vi "Import File - Tx Packet XML.vi"(6 "Root Node":refnum<k24>, 8 "error in (no error)":errorcluster) -> (0 "error out":errorcluster, 1 "Packet Header Data":T6, 4 "Tx Packet":T1 {"Endianness" items=["big-endian"=0, "little-endian"=2]})   [LabVIEW 2016, in "UDP-Custom-Device System Explorer.lvlib"]
uses:
  UDP-Custom-Device System Explorer.lvlib
  System.Xml
  Types/XML - New/ImpExp - Packet Headers.ctl
  Types/XML - New/ImpExp - Tx Packet Data.ctl
  <vilib>/NI Veristand/Custom Device API/Custom Device Item Info.ctl
  Shared/Types/Shared - Channel Data Type.ctl
  Shared/Types/Shared - Buffered.PacketInfo.ctl
  Shared/Types/Shared - Pointer Encoding.ctl
  <vilib>/NI VeriStand/Custom Device API/Custom Device API.lvlib
  Shared/UDP-Custom-Device Shared.lvlib
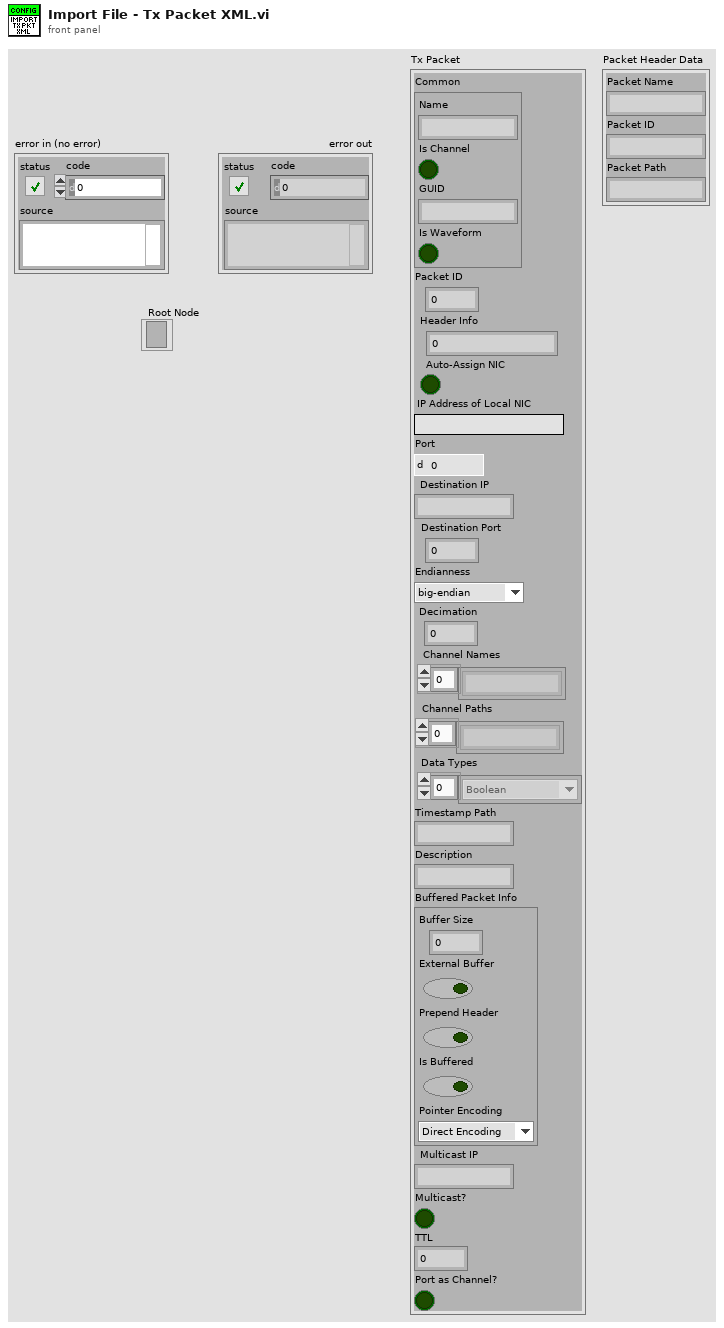
[diagram p1: front panel]
types:
  T1 = typedef "UDP-Custom-Device System Explorer.lvlib/ImpExp - Tx Packet Data.ctl" = cluster{"Common":T2, "Packet ID":i32, "Header Info":u32, "Auto-Assign NIC":bool, "IP Address of Local NIC":string, "Port":u16, "Destination IP":string, "Destination Port":u16, "Endianness":u16, "Decimation":u16, "Channel Names":string[], "Channel Paths":string[], "Data Types":T3[], "Timestamp Path":string, "Description":string, "Buffered Packet Info":T4, "Multicast IP":string, "Multicast?":bool, "TTL":u16, "Port as Channel?":bool}
  T2 = typedef "Custom Device API.lvlib/Custom Device Item Info.ctl" = cluster{"Name":string, "Is Channel":bool, "GUID":string, "Is Waveform":bool}
  T3 = typedef "UDP-Custom-Device Shared.lvlib/Shared - Channel Data Type.ctl" = enum16{"Boolean", "Single", "Double", "I8", "I16", "I32", "I64", "U8", "U16", "U32", "U64"}
  T4 = typedef "UDP-Custom-Device Shared.lvlib/Shared - Buffered.PacketInfo.ctl" = cluster{"Buffer Size":i32, "External Buffer":bool, "Prepend Header":bool, "Is Buffered":bool, "Pointer Encoding":T5}
  T5 = typedef "UDP-Custom-Device Shared.lvlib/Shared - Pointer Encoding.ctl" = enum16{"Direct Encoding", "Conversion Encoding"}
  T6 = typedef "UDP-Custom-Device System Explorer.lvlib/ImpExp - Packet Headers.ctl" = cluster{"Packet Name":string, "Packet ID":string, "Packet Path":string}
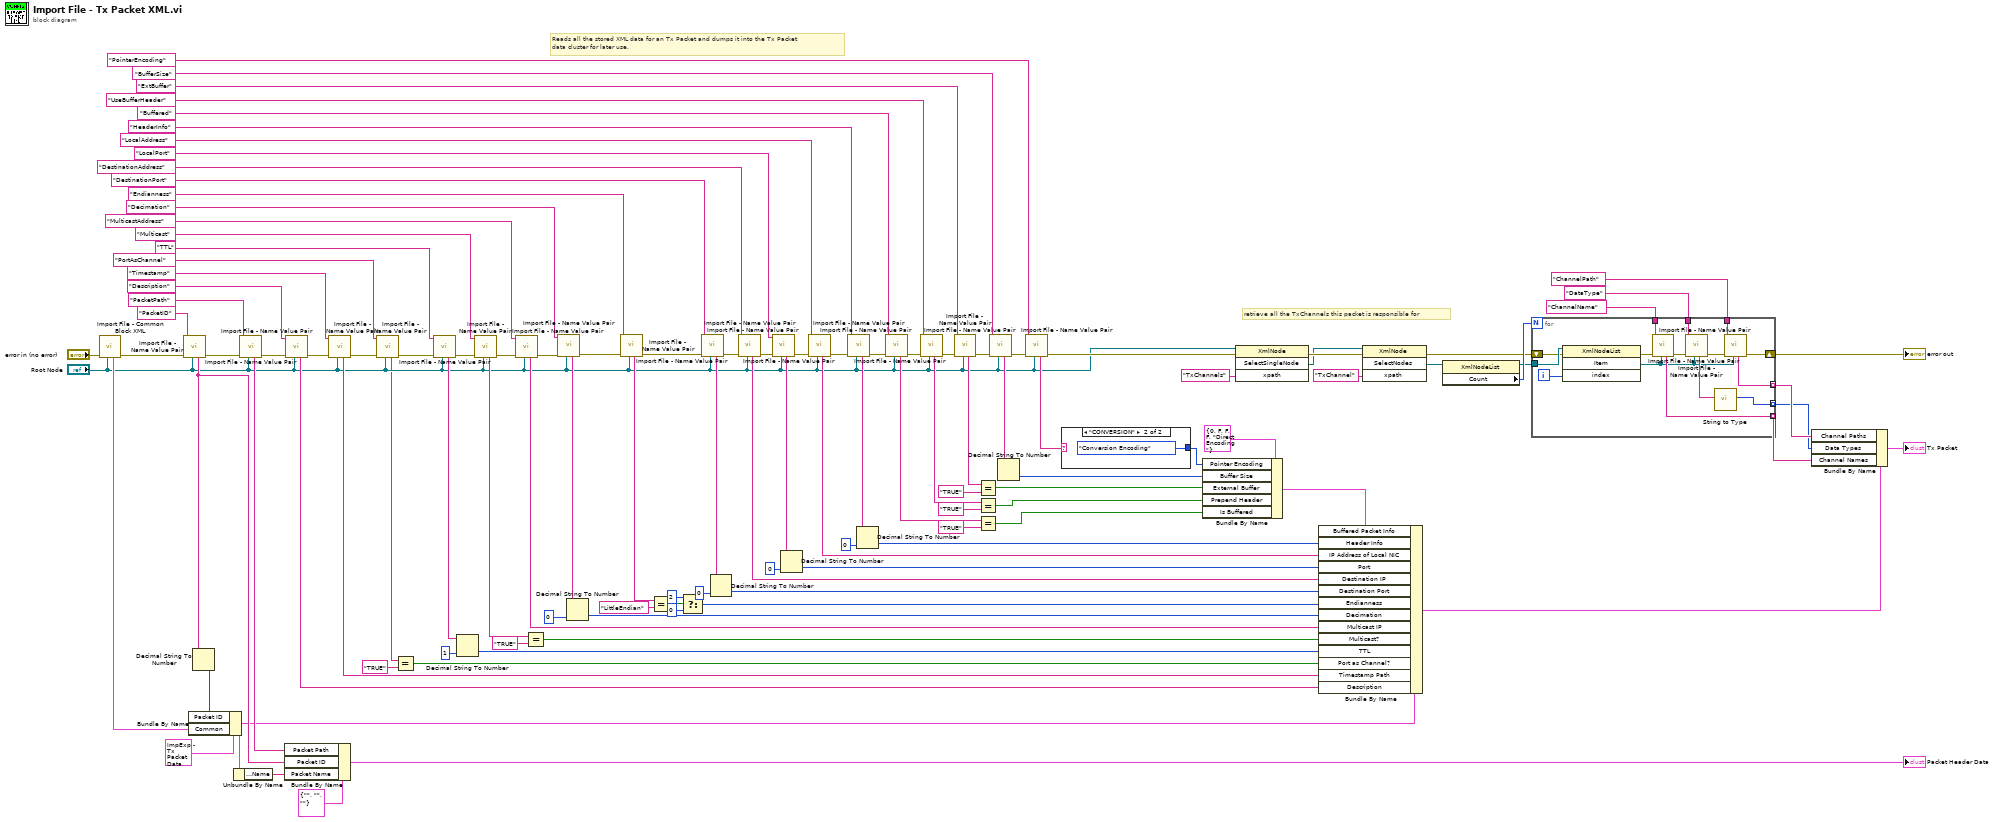
[diagram p0: block diagram]
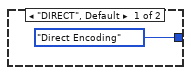
[diagram p2: hidden frame]
diagram:
  # "Reads all the stored XML data for an Tx Packet and dumps it into the Tx Packet\ndata cluster for later use."
  # "retrieve all the TxChannels this packet is responsible for"
  n1 = call "Import File - Common Block XML.vi"("Root Node"="Root Node", "error in (no error)"="error in (no error)") -> ("error out"=w110:errorcluster, "Common"=w114:T2)  [unwired: 8 in]
  n2 = call "Import File - Name Value Pair.vi"("Root Node"="Root Node", "error in (no error)"=w110, "Node Name"="PacketID") -> ("error out"=w107:errorcluster, "Value"=w105:string)  [unwired: 7 in]
  n3 = Decimal String To Number(string=w105) -> (number=w106:i32)  [unwired: 2 in, 1 out]
  n4 = Bundle By Name(cluster=T1 {"Common"={"Name"="", "Is Channel"=FALSE, "GUID"="", "Is Waveform"=FALSE}, "Packet ID"=0, "Header Info"=0, "Auto-Assign NIC"=FALSE, "IP Address of Local NIC"="", "Port"=0, "Destination IP"="", "Destination Port"=0, "Endianness"=0, "Decimation"=0, "Channel Names"=[], "Channel Paths"=[], "Data Types"=[], "Timestamp Path"="", "Description"="", "Buffered Packet Info"={"Buffer Size"=0, "External Buffer"=FALSE, "Prepend Header"=FALSE, "Is Buffered"=FALSE, "Pointer Encoding"=enum."Direct Encoding"}, "Multicast IP"="", "Multicast?"=FALSE, "TTL"=0, "Port as Channel?"=FALSE} ("Tx Packet"), "Packet ID"=w106, "Common"=w114) -> (w103:T1)
  n5 = Unbundle By Name(w103) -> ("Common.Name"=w112:string)
  n6 = call "Import File - Name Value Pair.vi"("Root Node"="Root Node", "error in (no error)"=w107, "Node Name"="PacketPath") -> ("error out"=w102:errorcluster, "Value"=w104:string)  [unwired: 7 in]
  n7 = Bundle By Name(cluster=T6 {"Packet Name"="", "Packet ID"="", "Packet Path"=""} ("Packet Header Data"), "Packet Path"=w104, "Packet ID"=w105, "Packet Name"=w112) -> (→"Packet Header Data":T6)
  n8 = call "Import File - Name Value Pair.vi"("Root Node"="Root Node", "error in (no error)"=w102, "Node Name"="Description") -> ("error out"=w100:errorcluster, "Value"=w86:string)  [unwired: 7 in]
  n9 = call "Import File - Name Value Pair.vi"("Root Node"="Root Node", "error in (no error)"=w100, "Node Name"="Timestamp") -> ("error out"=w6:errorcluster, "Value"=w85:string)  [unwired: 7 in]
  n10 = call "Import File - Name Value Pair.vi"("Root Node"="Root Node", "error in (no error)"=w6, "Node Name"="PortAsChannel" ("Tag Name")) -> ("error out"=w7:errorcluster, "Value"=w2:string)  [unwired: 7 in]
  n11 = Equal?(x=w2, y="TRUE") -> (x = y?=w1:bool)
  n12 = call "Import File - Name Value Pair.vi"("Root Node"="Root Node", "error in (no error)"=w7, "Node Name"="TTL" ("Tag Name")) -> ("error out"=w24:errorcluster, "Value"=w14:string)  [unwired: 7 in]
  n13 = Decimal String To Number(string=w14, default (0L)=u16 1 ("default (0 I32)")) -> (number=w13:u16)  [unwired: 1 in, 1 out]
  n14 = call "Import File - Name Value Pair.vi"("Root Node"="Root Node", "error in (no error)"=w24, "Node Name"="Multicast" ("Tag Name")) -> ("error out"=w25:errorcluster, "Value"=w17:string)  [unwired: 7 in]
  n15 = call "Import File - Name Value Pair.vi"("Root Node"="Root Node", "error in (no error)"=w25, "Node Name"="MulticastAddress" ("Tag Name")) -> ("error out"=w23:errorcluster, "Value"=w19:string)  [unwired: 7 in]
  n16 = Equal?(x=w17, y="TRUE") -> (x = y?=w16:bool)
  n17 = call "Import File - Name Value Pair.vi"("Root Node"="Root Node", "error in (no error)"=w23, "Node Name"="Decimation") -> ("error out"=w72:errorcluster, "Value"=w73:string)  [unwired: 7 in]
  n18 = Decimal String To Number(string=w73, default (0L)=u16 0 ("Decimation")) -> (number=w75:u16)  [unwired: 1 in, 1 out]
  n19 = call "Import File - Name Value Pair.vi"("Root Node"="Root Node", "error in (no error)"=w72, "Node Name"="Endianness") -> ("error out"=w71:errorcluster, "Value"=w67:string)  [unwired: 7 in]
  n20 = Equal?(x=w67, y="LittleEndian") -> (x = y?=w69:bool)
  n21 = Select(t=u16 2 ("Endianness"), s=w69, f=u16 0 ("Endianness")) -> (s? t:f=w65:u16)
  n22 = call "Import File - Name Value Pair.vi"("Root Node"="Root Node", "error in (no error)"=w71, "Node Name"="DestinationPort") -> ("error out"=w96:errorcluster, "Value"=w63:string)  [unwired: 7 in]
  n23 = Decimal String To Number(string=w63, default (0L)=u16 0 ("default (0 I32)")) -> (number=w62:u16)  [unwired: 1 in, 1 out]
  n24 = call "Import File - Name Value Pair.vi"("Root Node"="Root Node", "error in (no error)"=w96, "Node Name"="DestinationAddress") -> ("error out"=w93:errorcluster, "Value"=w60:string)  [unwired: 7 in]
  n25 = call "Import File - Name Value Pair.vi"("Root Node"="Root Node", "error in (no error)"=w93, "Node Name"="LocalPort") -> ("error out"=w92:errorcluster, "Value"=w58:string)  [unwired: 7 in]
  n26 = Decimal String To Number(string=w58, default (0L)=u16 0 ("default (0 I32)")) -> (number=w57:u16)  [unwired: 1 in, 1 out]
  n27 = call "Import File - Name Value Pair.vi"("Root Node"="Root Node", "error in (no error)"=w92, "Node Name"="LocalAddress") -> ("error out"=w91:errorcluster, "Value"=w56:string)  [unwired: 7 in]
  n28 = call "Import File - Name Value Pair.vi"("Root Node"="Root Node", "error in (no error)"=w91, "Node Name"="HeaderInfo") -> ("error out"=w90:errorcluster, "Value"=w54:string)  [unwired: 7 in]
  n29 = Decimal String To Number(string=w54, default (0L)=u32 0 ("default (0 I32)")) -> (number=w53:u32)  [unwired: 1 in, 1 out]
  n30 = call "Import File - Name Value Pair.vi"("Root Node"="Root Node", "error in (no error)"=w90, "Node Name"="Buffered") -> ("error out"=w81:errorcluster, "Value"=w51:string)  [unwired: 7 in]
  n31 = call "Import File - Name Value Pair.vi"("Root Node"="Root Node", "error in (no error)"=w81, "Node Name"="UseBufferHeader") -> ("error out"=w80:errorcluster, "Value"=w48:string)  [unwired: 7 in]
  n32 = call "Import File - Name Value Pair.vi"("Root Node"="Root Node", "error in (no error)"=w80, "Node Name"="ExtBuffer") -> ("error out"=w79:errorcluster, "Value"=w47:string)  [unwired: 7 in]
  n33 = Equal?(x=w47, y="TRUE") -> (x = y?=w43:bool)
  n34 = Equal?(x=w48, y="TRUE") -> (x = y?=w44:bool)
  n35 = Equal?(x=w51, y="TRUE") -> (x = y?=w45:bool)
  n36 = call "Import File - Name Value Pair.vi"("Root Node"="Root Node", "error in (no error)"=w79, "Node Name"="BufferSize") -> ("error out"=w12:errorcluster, "Value"=w46:string)  [unwired: 7 in]
  n37 = Decimal String To Number(string=w46) -> (number=w42:i32)  [unwired: 2 in, 1 out]
  n38 = call "Import File - Name Value Pair.vi"("Root Node"="Root Node", "error in (no error)"=w12, "Node Name"="PointerEncoding" ("Tag Name")) -> ("error out"=w11:errorcluster, "Value"=w8:string)  [unwired: 7 in]
  n39 = case shown="\"CONVERSION\"" w8 {
    tunnel: [Shared_-_Pointer_Encoding."Direct Encoding" ("Pointer Encoding") Shared_-_Pointer_Encoding."Conversion Encoding" ("Pointer Encoding")] -> w9
    frame "DIRECT", Default {
    }
    frame "CONVERSION" {
    }
  }
  n40 = Bundle By Name(cluster=T4 {"Buffer Size"=0, "External Buffer"=FALSE, "Prepend Header"=FALSE, "Is Buffered"=FALSE, "Pointer Encoding"=enum."Direct Encoding"} ("Buffered Packet Info"), "Pointer Encoding"=w9, "Buffer Size"=w42, "External Buffer"=w43, "Prepend Header"=w44, "Is Buffered"=w45) -> (w83:T4)
  n41 = invoke class="XmlNode" method="SelectSingleNode"(reference="Root Node", error in=w11, "xpath"="TxChannels") -> (error out=w41:errorcluster, "SelectSingleNode"=w40:refnum<k24>)  [unwired: 1 in, 2 out]
  n42 = Bundle By Name(cluster=w103, "Buffered Packet Info"=w83, "Header Info"=w53, "IP Address of Local NIC"=w56, "Port"=w57, "Destination IP"=w60, "Destination Port"=w62, "Endianness"=w65, "Decimation"=w75, "Multicast IP"=w19, "Multicast?"=w16, "TTL"=w13, "Port as Channel?"=w1, "Timestamp Path"=w85, "Description"=w86) -> (w82:T1)
  n43 = invoke class="XmlNode" method="SelectNodes"(reference=w40, error in=w41, "xpath"="TxChannel") -> (error out=w33:errorcluster, "SelectNodes"=w38:refnum<k24>)  [unwired: 1 in, 2 out]
  n44 = property class="XmlNodeList"(reference=w38) -> (reference out=w32:refnum<k24>, "Count"=w34:i32)  [unwired: 1 in, 1 out]
  n45 = for {
    N: w34 -> [_]
    shift-right: [w122] -> w26
    shift-left: w33 -> [w132]
    tunnel: w32 -> [w133]
    tunnel: "ChannelName" ("xpath") -> [w128]
    tunnel: "DataType" ("xpath") -> [w127]
    tunnel: [w126] -> w28 mode=indexing
    tunnel: [w124] -> w29 mode=indexing
    tunnel: "ChannelPath" ("xpath") -> [w121]
    tunnel: [w119] -> w30 mode=indexing
    i -> [w131]
    n46 = invoke class="XmlNodeList" method="Item"(reference=w133, error in=w132, "index"=w131) -> (error out=w130:errorcluster, "Item"=w120:refnum<k24>)  [unwired: 1 in, 2 out]
    n47 = call "Import File - Name Value Pair.vi"("Root Node"=w120, "error in (no error)"=w130, "Node Name"=w128) -> ("error out"=w129:errorcluster, "Value"=w126:string)  [unwired: 7 in]
    n48 = call "Import File - Name Value Pair.vi"("Root Node"=w120, "error in (no error)"=w129, "Node Name"=w127) -> ("error out"=w123:errorcluster, "Value"=w125:string)  [unwired: 7 in]
    n49 = call "String to Type.vi"("String Type"=w125) -> ("Data Type"=w124:T3)  [unwired: 10 in]
    n50 = call "Import File - Name Value Pair.vi"("Root Node"=w120, "error in (no error)"=w123, "Node Name"=w121) -> ("error out"=w122:errorcluster, "Value"=w119:string)  [unwired: 7 in]
  }
  "error out" <- w26
  n51 = Bundle By Name(cluster=w82, "Channel Paths"=w30, "Data Types"=w29, "Channel Names"=w28) -> (→"Tx Packet":T1)
